vi "Launcher.vi"() -> ()   [LabVIEW 2020]
uses:
  <vilib>/ActorFramework/Message Enqueuer/Message Enqueuer.lvclass
  Generador Funciones/Generador Funciones/Generador Funciones.lvclass
  C:/Program Files (x86)/National Instruments/LabVIEW 2020/vi.lib/ActorFramework/Actor/Actor.lvclass
  Contador Binario/Contador Binario/Contador Binario.lvclass
  <vilib>/ActorFramework/Message Enqueuer/Message Enqueuer.lvclass/Message Enqueuer.ctl
  <vilib>/ActorFramework/Message Enqueuer/Enqueue.vi
  <vilib>/ActorFramework/Stop Msg/Stop Msg.lvclass
  C:/Program Files (x86)/National Instruments/LabVIEW 2020/vi.lib/ActorFramework/Message/Message.lvclass
  <vilib>/ActorFramework/Message Priority Queue/Priority Enqueue.vi
  <vilib>/ActorFramework/Actor/Actor.lvclass
panel:
  in  "Exit":bool
  in  "Counter":u16(ring)
  in  "Add Button":bool
  in  "stop":bool
  in  "Type":enum16{"Generador", "Binario"}(ring)
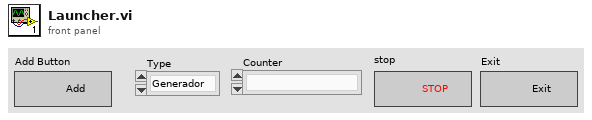
[diagram p1: front panel]
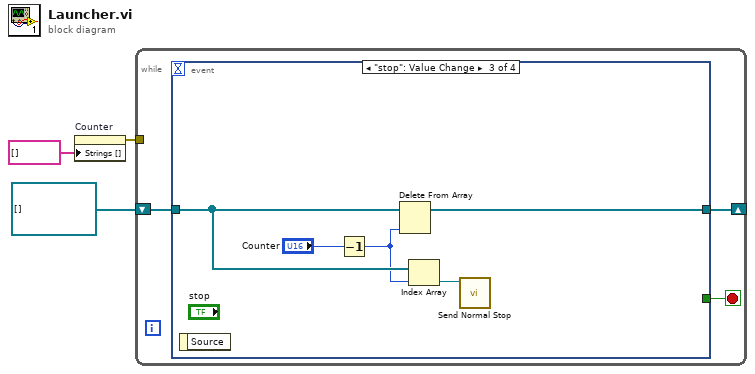
[diagram p0: block diagram]
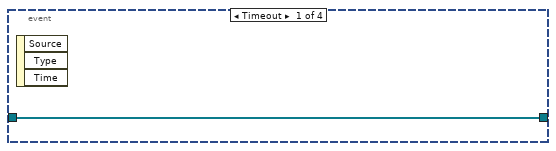
[diagram p2: hidden frame]
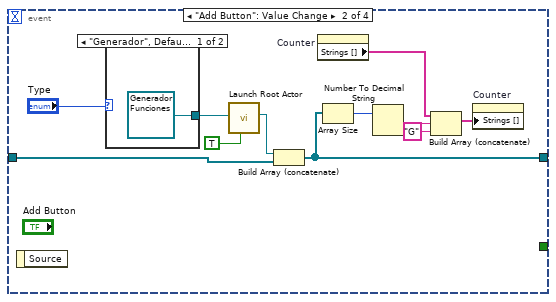
[diagram p3: hidden frame]
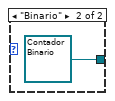
[diagram p4: hidden frame]
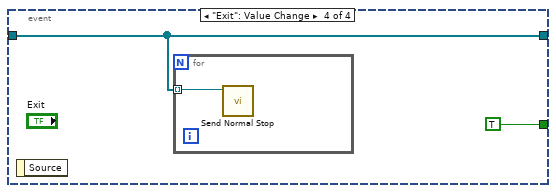
[diagram p5: hidden frame]
diagram:
  n1 = property on="Counter" class="Ring (strict)"("Strings []"=string[] []) -> (error out=w2:errorcluster)  [unwired: 2 in, 1 out]
  n2 = while {
    tunnel: w2 -> [_]
    shift-right: [w5] -> _
    shift-left: refnum<class "Message Enqueuer.lvclass">[] [] -> [w6]
    stop <- w4 stop-if-true
    n3 = event shown="[2] \"stop\": Value Change" {
      selector: _ -> [_ _ _ _]
      dyn-events: _ -> [_ _ _ _]
      timeout: _ -> [_ _ _ _]
      tunnel: w6 -> [w7 w14 w24 w26]
      tunnel: [w7 w12 w21 w26] -> w5
      tunnel: [_ _ _ TRUE] -> w4
      event Timeout {
        n4 = event-data() -> ()  [unwired: 1 in, 3 out]
      }
      event "Add Button": Value Change {
        n5 = event-data() -> ()  [unwired: 1 in, 1 out]
        n6 = case shown="\"Generador\", Default" "Type" {
          tunnel: [refnum<class "Generador Funciones.lvclass"> refnum ("Generador Funciones.lvlib:Generador Funciones.lvclass") refnum<class "Contador Binario.lvclass"> refnum ("Contador Binario.lvlib:Contador Binario.lvclass")] -> w13
          frame "Generador", Default {
          }
          frame "Binario" {
          }
        }
        n7 = call <vilib>:"Launch Root Actor.vi"("Open Actor Core front panel? (F)"=TRUE, "Actor"=w13) -> ("Actor's Enqueuer"=w16:refnum<class "Message Enqueuer.lvclass">)  [unwired: 8 in, 1 out]
        n8 = Build Array (concatenate) "Build Array"(w16, w14) -> (w12:refnum<class "Message Enqueuer.lvclass">[])
        n9 = property on="Counter" class="Ring (strict)"() -> ("Strings []"=w10:string[])  [unwired: 2 in, 2 out]
        n10 = Array Size(array=w12) -> (size(s)=w17:i32)
        n11 = Number To Decimal String(number=w17) -> (decimal integer string=w18:string)  [unwired: 1 in]
        n12 = Build Array (concatenate)(w10, w18, "G" ("element")) -> (w15:string[])
        n13 = property on="Counter" class="Ring (strict)"("Strings []"=w15) -> ()  [unwired: 2 in, 2 out]
      }
      event "stop": Value Change {
        n14 = event-data() -> ()  [unwired: 1 in, 1 out]
        n15 = Decrement(x="Counter") -> (x-1=w22:u16)
        n16 = Delete From Array(array=w24, index=w22) -> (array with subset deleted=w21:refnum<class "Message Enqueuer.lvclass">[])  [unwired: 1 in, 1 out]
        n17 = Index Array "Index Array"(array=w24, index=w22) -> (element=w23:refnum<class "Message Enqueuer.lvclass">)
        n18 = call <vilib>:"Send Normal Stop.vi"("Message Enqueuer"=w23) -> ()  [unwired: 10 in, 1 out]
      }
      event "Exit": Value Change {
        n19 = event-data() -> ()  [unwired: 1 in, 1 out]
        n20 = for {
          tunnel: w26 -> [w28] mode=indexing
          n21 = call <vilib>:"Send Normal Stop.vi"("Message Enqueuer"=w28) -> ()  [unwired: 10 in, 1 out]
        }
      }
    }
  }
